vi "Parse Params.vi"(8 "error in (no error)":errorcluster, 9 "{JSON} Params":string, 11 "JSON-RPC in":refnum<class "JSON-RPC.lvclass">) -> (0 "error out":errorcluster, 1 "Params":string[](array[string]), 2 "Names":string[](array[string]), 3 "JSON-RPC out":refnum<class "JSON-RPC.lvclass">)   [LabVIEW 2019, in "JSON-RPC.lvclass"]
uses:
  JSON-RPC.lvclass
  <vilib>/JDP Science/JSONtext/Get Array Elements.vi
  <vilib>/JDP Science/JSONtext/Get all Object Items.vi
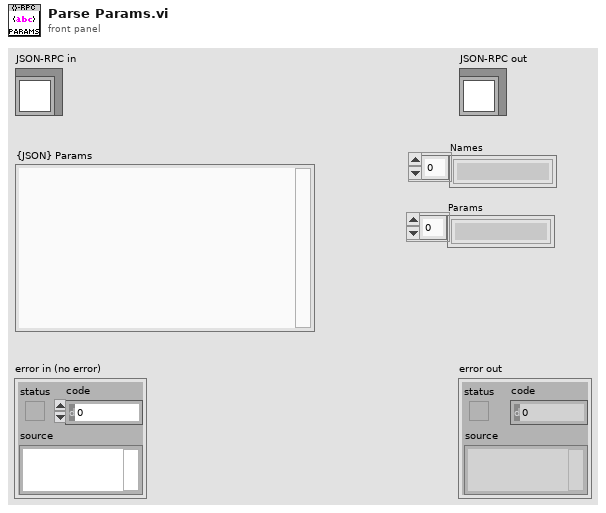
[diagram p1: front panel]
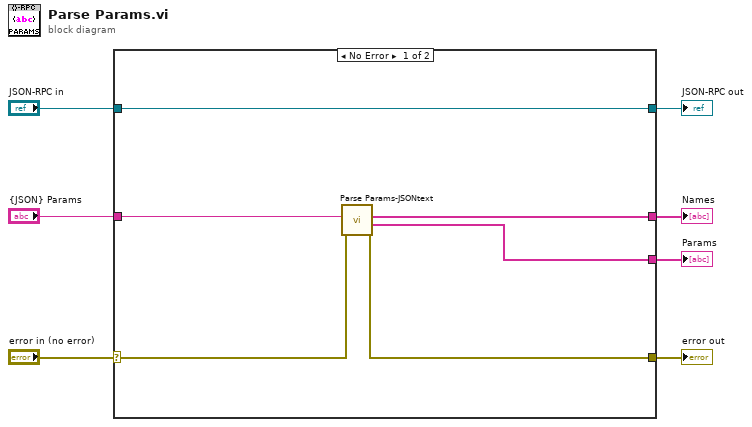
[diagram p0: block diagram]
diagram:
  n1 = case shown="No Error" "error in (no error)" {
    selector: "error in (no error)" -> [w12 w15]
    tunnel: [w11 w15] -> w6
    tunnel: [w8 w14] -> w4
    tunnel: "JSON-RPC in" -> [w8 w14]
    tunnel: "{JSON} Params" -> [w13 _]
    tunnel: [w10 _] -> w1
    tunnel: [w9 _] -> w2
    frame No Error {
      n2 = call "Parse Params-JSONtext.vi"("error in (no error)"=w12, "JSON"=w13) -> ("error out"=w11:errorcluster, "Params"=w10:string[], "Names"=w9:string[])  [unwired: 7 in]
    }
    frame Error {
    }
  }
  "error out" <- w6
  "JSON-RPC out" <- w4
  "Names" <- w2
  "Params" <- w1
